vi "Convert Database Variant to Data.vi"() -> ()   [LabVIEW 2013]
doc: "The example demonstrates how to convert database variants that you read from a database to an appropriate LabVIEW data type. For example you can convert a 1D array of database variants to a cluster of LabVIEW data. This example reads data from a predefined database, located at LabVIEW\\examples\\database\\LabVIEW.mdb, and uses the Database Variant To Data function to do the conversion. Examine the block diagram of this example VI for more information about using this function."
uses:
  Connection.llb/DB Tools Open Connec (Path).vi
  _DB Variant To Data/Database Variant To Data.xnode
  NI_Database_API_64.lvlib
panel:
  in  "Tab Control":T1(tab)=enum."2DArrayto1DArrayofCluster"
  out "one row":cluster{i32, string, string, string}
  out "one column":string[](array[string])
  out "all data":cluster{i32, string, string, string}[](array[cluster])
  out "all data as String":string[][](array[string])
  in  "GO Button":bool
  # "INSTRUCTIONS:\n\nSelect the type of variant you want to convert and click the GO button to execute."
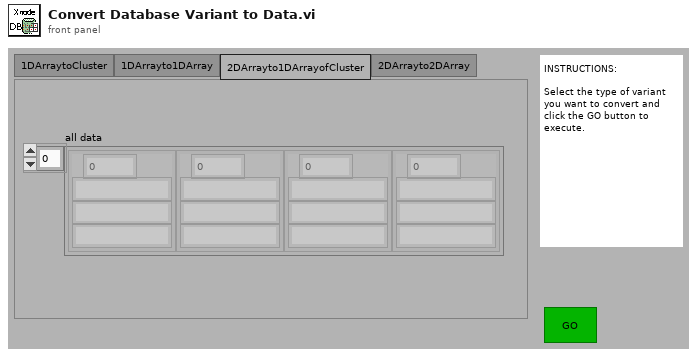
[diagram p1: front panel]
types:
  T1 = enum32{"1DArraytoCluster", "1DArrayto1DArray", "2DArrayto1DArrayofCluster", "2DArrayto2DArray"}
  T2 = typedef "NI_Database_API_64.lvlib/Conn ObjectReference.ctl" = refnum<k1>
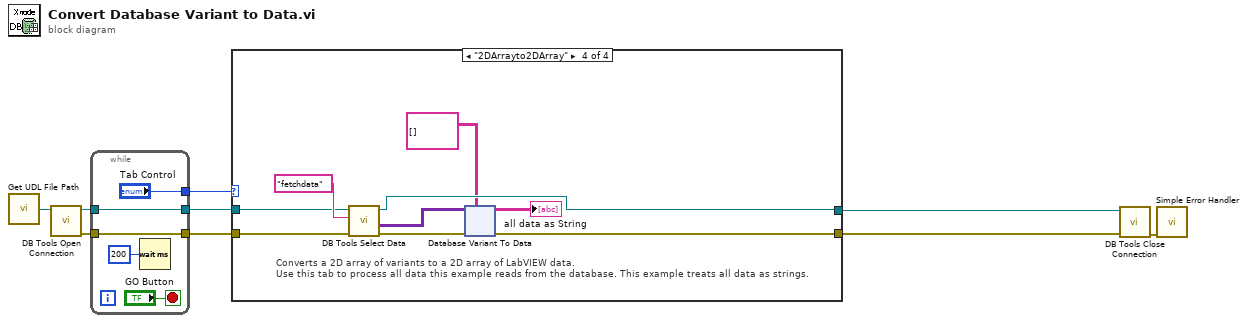
[diagram p0: block diagram]
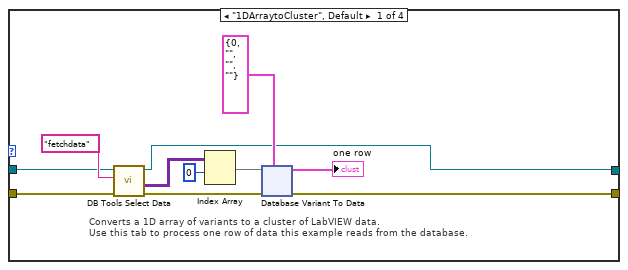
[diagram p2: hidden frame]
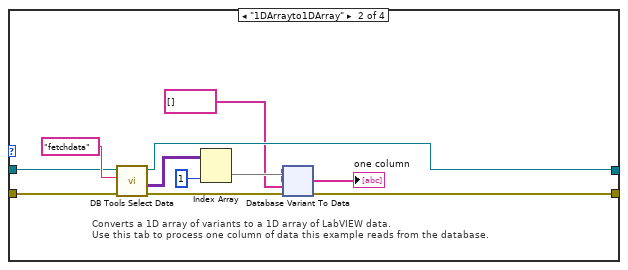
[diagram p3: hidden frame]
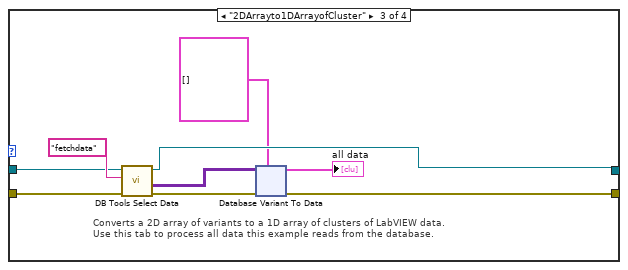
[diagram p4: hidden frame]
diagram:
  n1 = call "Get UDL File Path.vi"() -> ("UDL file path"=w6:path)  [unwired: 1 in]
  n2 = call-poly "DB Tools Open Connection.vi"("connection information"=w6) -> ("error out"=w8:errorcluster, "connection reference"=w9:T2)  [unwired: 7 in]
  n3 = while {
    tunnel: ["Tab Control"] -> w5
    tunnel: [w12] -> w4
    tunnel: w9 -> [w12]
    tunnel: w8 -> [w11]
    tunnel: [w11] -> w3
    stop <- "GO Button" stop-if-true
    n4 = Wait (ms)(milliseconds to wait=u32 200) -> ()  [unwired: 1 out]
  }
  n5 = case shown="\"2DArrayto2DArray\"" w5 {
    tunnel: w4 -> [w23 w160 w209 w350]
    tunnel: w3 -> [w22 w159 w208 w351]
    tunnel: [w18 w157 w206 w349] -> w2
    tunnel: [w16 w158 w207 w348] -> w1
    frame "1DArraytoCluster", Default {
      # "Converts a 1D array of variants to a cluster of LabVIEW data.\nUse this tab to process one row of data this example reads from the database."
      n6 = call "DB Tools Select Data.vi"("error in (no error)"=w22, "table"="fetchdata", "connection reference"=w23) -> ("error out"=w17:errorcluster, "data"=w21:variant[][], "connection reference out"=w18:T2)  [unwired: 3 in]
      n7 = Index Array(array=w21, index (row)=0) -> (element=w24:variant[])  [unwired: 1 in]
      n8 = xnode "Database Variant To Data"("database variant"=w24, "error in"=w17, "type"=cluster{i32, string, string, string} {0, "", "", ""}) -> ("data"=→"one row":cluster{i32, string, string, string}, "error out"=w16:errorcluster)
    }
    frame "1DArrayto1DArray" {
      # "Converts a 1D array of variants to a 1D array of LabVIEW data. \nUse this tab to process one column of data this example reads from the database."
      n9 = call "DB Tools Select Data.vi"("error in (no error)"=w159, "table"="fetchdata", "connection reference"=w160) -> ("error out"=w161:errorcluster, "data"=w162:variant[][], "connection reference out"=w157:T2)  [unwired: 3 in]
      n10 = Index Array(array=w162, index (col)=1 ("index (row)")) -> (element=w163:variant[])  [unwired: 1 in]
      n11 = xnode "Database Variant To Data"("database variant"=w163, "error in"=w161, "type"=string[] []) -> ("data"=→"one column":string[], "error out"=w158:errorcluster)
    }
    frame "2DArrayto1DArrayofCluster" {
      # "Converts a 2D array of variants to a 1D array of clusters of LabVIEW data.\nUse this tab to process all data this example reads from the database."
      n12 = call "DB Tools Select Data.vi"("error in (no error)"=w208, "table"="fetchdata", "connection reference"=w209) -> ("error out"=w210:errorcluster, "data"=w204:variant[][], "connection reference out"=w206:T2)  [unwired: 3 in]
      n13 = xnode "Database Variant To Data"("database variant"=w204, "error in"=w210, "type"=cluster{i32, string, string, string}[] []) -> ("data"=→"all data":cluster{i32, string, string, string}[], "error out"=w207:errorcluster)
    }
    frame "2DArrayto2DArray" {
      # "Converts a 2D array of variants to a 2D array of LabVIEW data. \nUse this tab to process all data this example reads from the database. This example treats all data as strings."
      n14 = call "DB Tools Select Data.vi"("error in (no error)"=w351, "table"="fetchdata", "connection reference"=w350) -> ("error out"=w353:errorcluster, "data"=w352:variant[][], "connection reference out"=w349:T2)  [unwired: 3 in]
      n15 = xnode "Database Variant To Data"("database variant"=w352, "error in"=w353, "type"=string[][] []) -> ("data"=→"all data as String":string[][], "error out"=w348:errorcluster)
    }
  }
  n16 = call "DB Tools Close Connection.vi"("error in (no error)"=w1, "connection reference"=w2) -> ("error out"=w7:errorcluster)  [unwired: 5 in]
  n17 = call <vilib>:"Simple Error Handler.vi"("error in (no error)"=w7) -> ()  [unwired: 4 in, 5 out]
